vi "Reset Plain Formatting.vi"(8 "error in (no error)":errorcluster, 11 "String Ref":refnum<vi>) -> (0 "error out":errorcluster, 3 "String Ref out":refnum<vi>)   [LabVIEW 2020, in "VI Properties Editor.lvlib"]
doc: "Finds where the formatting of the text of <B>Str Ref</B> is bold."
uses:
  VI Properties Editor.lvlib
  <vilib>/Utility/miscctls.llb/LVSelectionTypeDef.ctl
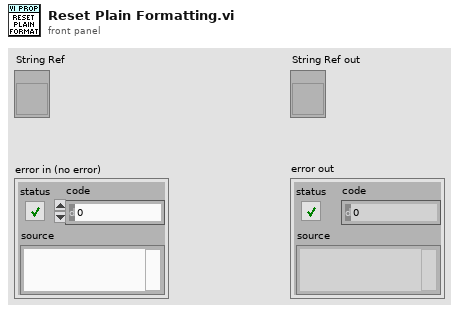
[diagram p1: front panel]
types:
  T1 = typedef "LVSelectionTypeDef.ctl" = cluster{"Selection Start":u32, "Selection End":u32}
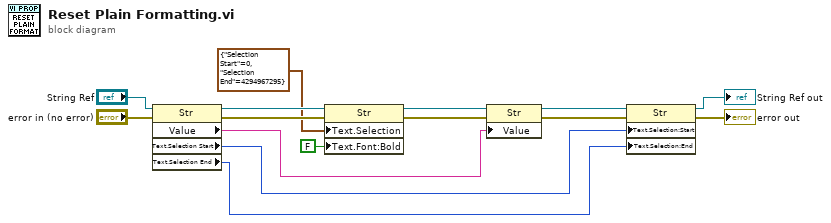
[diagram p0: block diagram]
diagram:
  n1 = property class="Str"(reference="String Ref", error in="error in (no error)") -> (reference out=w15:refnum<vi>, error out=w14:errorcluster, "Value"=w1:string, "Text.Selection Start"=w9:u32, "Text.Selection End"=w10:u32)
  n2 = property on="Property Node" class="Str"(reference=w15, error in=w14, "Text.Selection"=T1 {"Selection Start"=0, "Selection End"=4294967295}, "Text.Font:Bold"=FALSE) -> (reference out=w3:refnum<vi>, error out=w12:errorcluster)
  n3 = property class="Str"(reference=w3, error in=w12, "Value"=w1) -> (reference out=w2:refnum<vi>, error out=w4:errorcluster)
  n4 = property on="Property Node" class="Str"(reference=w2, error in=w4, "Text.Selection:Start"=w9, "Text.Selection:End"=w10) -> (reference out=→"String Ref out":refnum<vi>, error out=→"error out":errorcluster)
